vi "ExposeLogCallback.vi"(4 "Callback Info":T1, 5 "Event Data":cluster{"sender":refnum<k24>, "e":refnum<k24>}, 6 "Control Ref":refnum<k24>, 7 "Event Common Data":T5) -> ()   [LabVIEW 2017]
uses:
  C:/Code/CMCryoSysCode/Expose/COM/CSCom/CSCom/bin/Release/CSCom.dll
  COM/CSCom/CSCom/bin/Release/CSCom.dll
  ExposeMessageCallbackInfo.ctl
  ExposeInfo.ctl
  ExposeHandlers.ctl
  ExposeMessageCallbackViRefrenceType.ctl
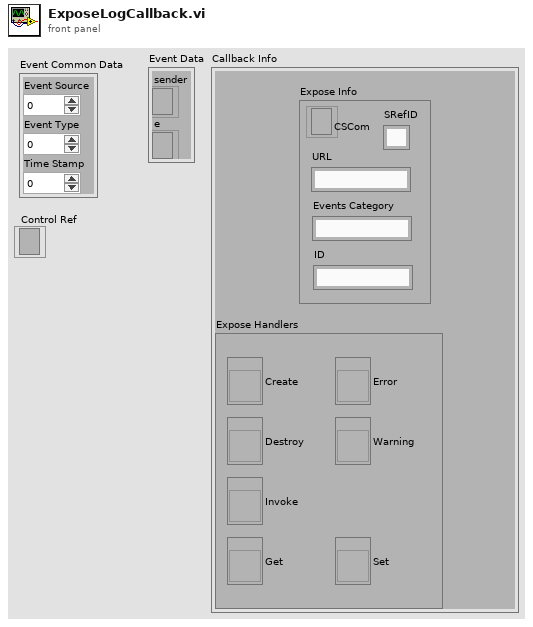
[diagram p1: front panel]
types:
  T1 = typedef "ExposeMessageCallbackInfo.ctl" = cluster{"Expose Info":T2, "Expose Handlers":T3}
  T2 = typedef "ExposeInfo.ctl" = cluster{"CSCom":refnum<k24>, "URL":string, "Events Category":string, "ID":string, "SRefID":string}
  T3 = typedef "ExposeHandlers.ctl" = cluster{"Create":T4, "Destroy":T4, "Invoke":T4, "Get":T4, "Set":T4, "Warning":T4, "Error":T4}
  T4 = typedef "ExposeMessageCallbackViRefrenceType.ctl" = refnum<vi>
  T5 = cluster{"Event Source":i32, "Event Type":u32, "Time Stamp":u32}
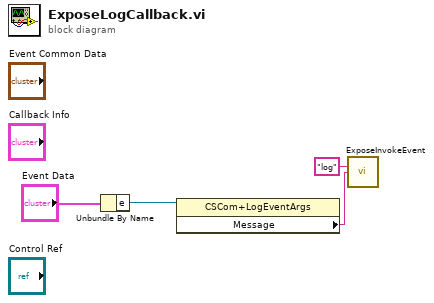
[diagram p0: block diagram]
diagram:
  n1 = Unbundle By Name("Event Data") -> ("e"=w3:refnum<k24>)
  n2 = property class="CSCom+LogEventArgs"(reference=w3) -> ("Message"=w2:string)  [unwired: 1 in, 2 out]
  n3 = call "ExposeInvokeEvent.vi"("name"="log", "Data"=w2) -> ()  [unwired: 13 in, 1 out]
